vi "Fetch Waveform.vi"(6 "Data Type":bool, 8 "error in (no error)":errorcluster, 9 "Timeout (5000 ms)":u32=5000, 10 "Channel (1: Channel 1)":u16(ring)=1 items=["Channel 1"=1, "Channel 2"=2, "Channel 3"=3, "Channel 4"=4], 11 "VISA resource name":refnum<visa-resource-name>) -> (0 "error out":errorcluster, 2 "Waveform Data":dbl[](graph), 3 "VISA resource name out":refnum<visa-resource-name>)   [LabVIEW 2015, in "ZhiYuan ZDS Series for TCP.lvlib"]
doc: "Returns the waveform the oscilloscope acquired for the specified channel. The waveform is from an acquisition that you initiate prior to calling this VI.\n\nYou use the Initiate VI to start an acquisition on the channels that you enable with the Configure Channel VI. The oscilloscope acquires waveforms for the enabled channels concurrently. You must call this VI separately for each enabled channel to obtain the waveforms.\n\nYou can call the Read Waveform VI instead of using low-level VIs.\n\n<B>Note:</B> Use this VI only with other low-level VIs. The high-level VIs automatically incorporate this functionality. This VI does not check the instrument status."
uses:
  ZhiYuan ZDS Series for TCP.lvlib
panel:
  # "Memory"
  # "Display"
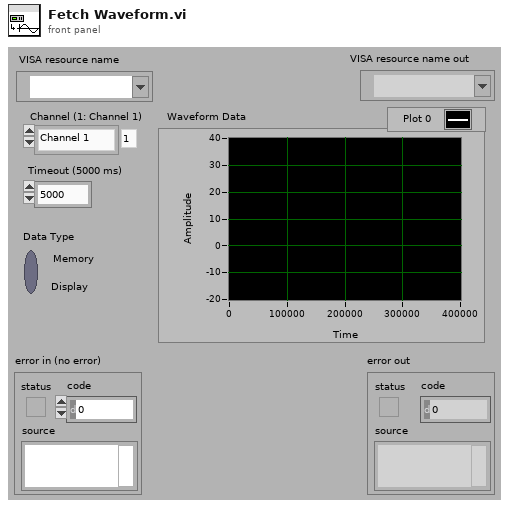
[diagram p1: front panel]
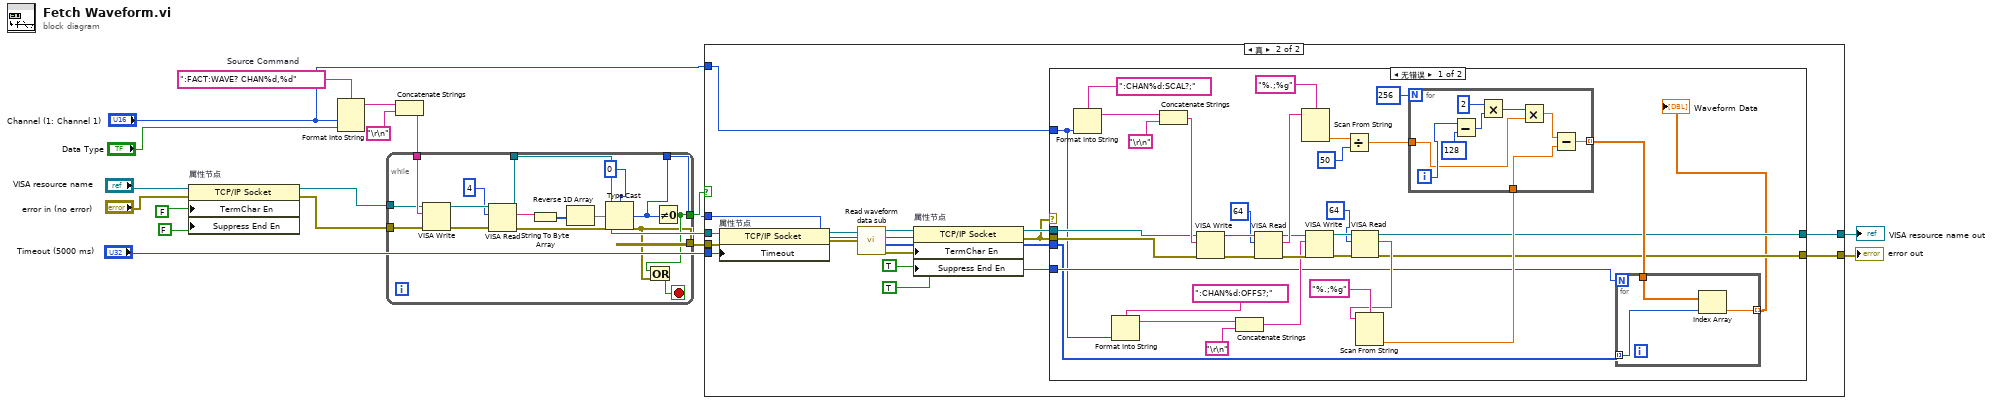
[diagram p0: block diagram]
diagram:
  w19 = ":FACT:WAVE? CHAN%d,%d"  # Source Command
  n1 = property on="属性节点" class="TCP/IP Socket"(reference="VISA resource name", error in="error in (no error)", "TermChar En"=FALSE, "Suppress End En"=FALSE ("Message Based Settings:Suppress End Enable")) -> (reference out=w5:refnum<visa-resource-name>, error out=w7:errorcluster)
  n2 = Format Into String(format string=w19, "Channel (1: Channel 1)", "Data Type") -> (resulting string=w17:string)  [unwired: 2 in, 1 out]
  n3 = Concatenate Strings(w17, "\r\n") -> (w6:string)
  n4 = while {
    tunnel: w7 -> [w34]
    tunnel: w6 -> [w33]
    tunnel: w5 -> [w32]
    tunnel: [w21] -> w4
    tunnel: [w29] -> w3
    tunnel: [w22] -> w2
    tunnel: [w23] -> w1
    stop <- w20 stop-if-true
    n5 = VISA Write(VISA resource name=w32, write buffer=w33, error in (no error)=w34) -> (VISA resource name out=w30:refnum<visa-resource-name>, error out=w31:errorcluster)  [unwired: 1 out]
    n6 = VISA Read(VISA resource name=w30, byte count=u32 4, error in (no error)=w31) -> (VISA resource name out=w29:refnum<visa-resource-name>, read buffer=w24:string, error out=w21:errorcluster)  [unwired: 1 out]
    n7 = String To Byte Array(string=w24) -> (unsigned byte array=w26:u8[])
    n8 = Reverse 1D Array(array=w26) -> (reversed array=w27:u8[])
    n9 = Type Cast(type=u32 0, x=w27) -> (*(type *) &x=w23:u32)
    n10 = Not Equal To 0?(x=w23) -> (x != 0?=w22:bool)
    n11 = Or(x=w22, y=w21) -> (x .or. y?=w20:bool)
  }
  n12 = case shown="真" w2 {
    tunnel: w3 -> [w35 w53]
    tunnel: w4 -> [w36 w52]
    tunnel: "Timeout (5000 ms)" -> [_ w50]
    tunnel: w1 -> [_ w49]
    tunnel: "Channel (1: Channel 1)" -> [_ w48]
    tunnel: [w35 w47] -> w13
    tunnel: [w36 w46] -> w12
    frame False {
    }
    frame True {
      n13 = property on="属性节点" class="TCP/IP Socket"(reference=w53, error in=w52, "Timeout"=w50) -> (reference out=w51:refnum<visa-resource-name>, error out=w40:errorcluster)
      n14 = call "Read waveform data sub.vi"("错误输入（无错误）"=w40, "读取数据大小"=w49, "VISA资源名称"=w51) -> ("错误输出"=w41:errorcluster, "波形数据"=w38:u8[], "返回数"=w39:u32, "VISA资源名称输出"=w42:refnum<visa-resource-name>)  [unwired: 3 in]
      n15 = property on="属性节点" class="TCP/IP Socket"(reference=w42, error in=w41, "TermChar En"=TRUE, "Suppress End En"=TRUE) -> (reference out=w43:refnum<visa-resource-name>, error out=w37:errorcluster)
      n16 = case shown="无错误" w37 {
        tunnel: w48 -> [w54 _]
        tunnel: [w61 w101] -> w47
        tunnel: [w60 w100] -> w46
        tunnel: w43 -> [w58 w101]
        tunnel: w37 -> [w57 w100]
        tunnel: w39 -> [w56 _]
        tunnel: w38 -> [w55 _]
        frame No Error {
          n17 = Format Into String(format string=":CHAN%d:SCAL?;", w54) -> (resulting string=w86:string)  [unwired: 2 in, 1 out]
          n18 = Format Into String(format string=":CHAN%d:OFFS?;", w54) -> (resulting string=w72:string)  [unwired: 2 in, 1 out]
          n19 = Concatenate Strings(w86, "\r\n") -> (w84:string)
          n20 = VISA Write(VISA resource name=w58, write buffer=w84, error in (no error)=w57) -> (VISA resource name out=w82:refnum<visa-resource-name>, error out=w83:errorcluster)  [unwired: 1 out]
          n21 = Concatenate Strings(w72, "\r\n") -> (w70:string)
          n22 = VISA Read(VISA resource name=w82, byte count=u32 64, error in (no error)=w83) -> (VISA resource name out=w78:refnum<visa-resource-name>, read buffer=w80:string, error out=w75:errorcluster)  [unwired: 1 out]
          n23 = Scan From String(format string="%.;%g", input string=w80) -> (output 1=w66:dbl)  [unwired: 3 in, 3 out]
          n24 = VISA Write(VISA resource name=w78, write buffer=w70, error in (no error)=w75) -> (VISA resource name out=w77:refnum<visa-resource-name>, error out=w74:errorcluster)  [unwired: 1 out]
          n25 = Divide(x=w66, y=50) -> (x/y=w64:dbl)
          n26 = VISA Read(VISA resource name=w77, byte count=u32 64, error in (no error)=w74) -> (VISA resource name out=w61:refnum<visa-resource-name>, read buffer=w68:string, error out=w60:errorcluster)  [unwired: 1 out]
          n27 = Scan From String(format string="%.;%g", input string=w68) -> (output 1=w63:dbl)  [unwired: 3 in, 3 out]
          n28 = for {
            N: 256 -> [_]
            tunnel: w64 -> [w94]
            tunnel: w63 -> [w92]
            tunnel: [w91] -> w62 mode=indexing
            i -> [w99]
            n29 = Subtract(x=w99, y=128) -> (x-y=w97:i32)
            n30 = Multiply(x=2, y=w97) -> (x*y=w95:i32)
            n31 = Multiply(x=w95, y=w94) -> (x*y=w93:dbl)
            n32 = Subtract(x=w93, y=w92) -> (x-y=w91:dbl)
          }
          n33 = for {
            N: w56 -> [_]
            tunnel: w62 -> [w90]
            tunnel: [w89] -> w59 mode=indexing
            tunnel: w55 -> [w88] mode=indexing
            n34 = Index Array(array=w90, index=w88) -> (element=w89:dbl)
          }
          "Waveform Data" <- w59
        }
        frame Error {
        }
      }
    }
  }
  "error out" <- w12
  "VISA resource name out" <- w13
